vi "Get Inertia Matrix.vi"(8 "error in (no error)":errorcluster, 11 "Link":refnum<class "NI_Robotics_Link.lvclass">) -> (0 "error out":errorcluster, 2 "Inertia Matrix":T1, 3 "Link 2":refnum<class "NI_Robotics_Link.lvclass">)   [LabVIEW 2017, in "NI_Robotics_Link.lvclass"]
uses:
  <vilib>/robotics/Kinematics/Link/NI_Robotics_Link.lvclass
  <vilib>/Analysis/Matrix/Datatypes/RealMatrix.ctl
  <vilib>/robotics/Kinematics/Link/NI_Robotics_Link.lvclass/NI_Robotics_Link.ctl
  <vilib>/Analysis/Matrix/NI_Matrix.lvlib
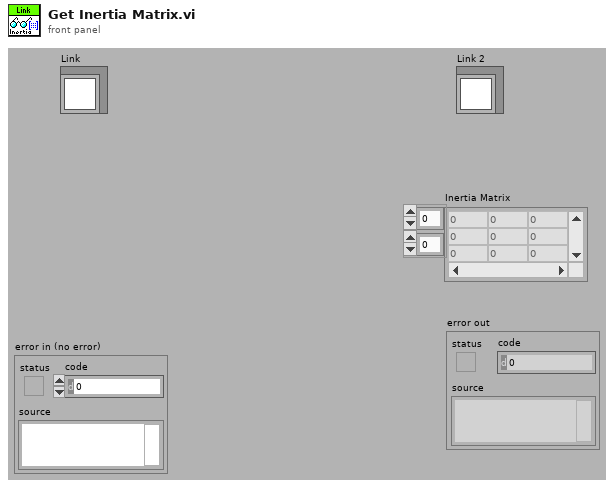
[diagram p1: front panel]
types:
  T1 = typedef "NI_Matrix.lvlib/RealMatrix.ctl" = dbl[][]
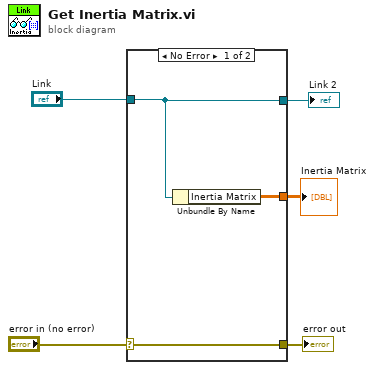
[diagram p0: block diagram]
diagram:
  n1 = case shown="No Error" "error in (no error)" {
    selector: "error in (no error)" -> [w6 w9]
    tunnel: "Link" -> [w7 w10]
    tunnel: [w8 _] -> w5
    tunnel: [w7 w10] -> w4
    tunnel: [w6 w9] -> w1
    frame No Error {
      n2 = Unbundle By Name(w7) -> ("Inertia Matrix"=w8:T1)
    }
    frame Error {
    }
  }
  "Link 2" <- w4
  "Inertia Matrix" <- w5
  "error out" <- w1
